vi "conv-var-vers-CONT.vi"(7 "Variable":string) -> (1 "Nature Var. (Ch)":string, 2 "Cont. ?":bool, 3 "Nature var.":T1)   [LabVIEW 2010, in "lv_04.lvlib"]
uses:
  lv_04.lvlib
  commandes/c_enum_nature_var.ctl
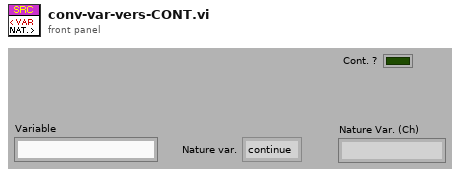
[diagram p1: front panel]
types:
  T1 = typedef "lv_04.lvlib/c_enum_nature_var.ctl" = enum16{"continue", "discrète"}
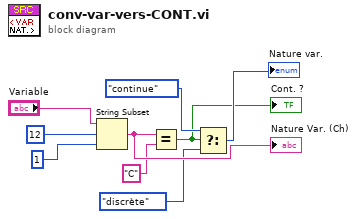
[diagram p0: block diagram]
diagram:
  n1 = String Subset(string="Variable", offset (0)=12, length (rest)=1 ("longueur (reste)")) -> (substring=w7:string)
  "Nature Var. (Ch)" <- w7
  n2 = Equal?(x=w7, y="C") -> (x = y?=w1:bool)
  "Cont. ?" <- w1
  n3 = Select(t=c_enum_nature_var."continue" ("Nature var."), s=w1, f=c_enum_nature_var."discrète" ("Nature var.")) -> (s? t:f=→"Nature var.":T1)
